vi "set units.vi"(8 "error in (no error)":errorcluster, 10 "Field Units (0: Gauss)":u16(ring) items=["Gauss", "Tesla", "Oersted", "Amp/meter"], 11 "VISA session":refnum<visa-resource-name>) -> (0 "error out":errorcluster, 3 "dup VISA session":refnum<visa-resource-name>)   [LabVIEW 2017]
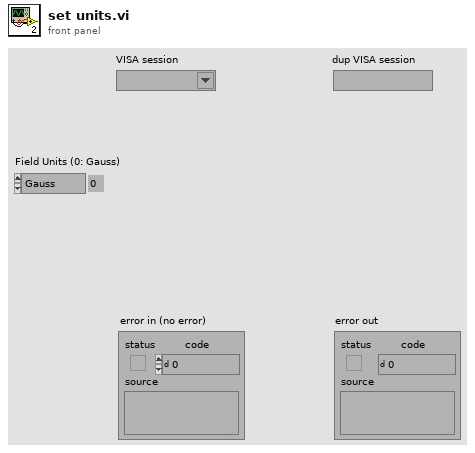
[diagram p1: front panel]
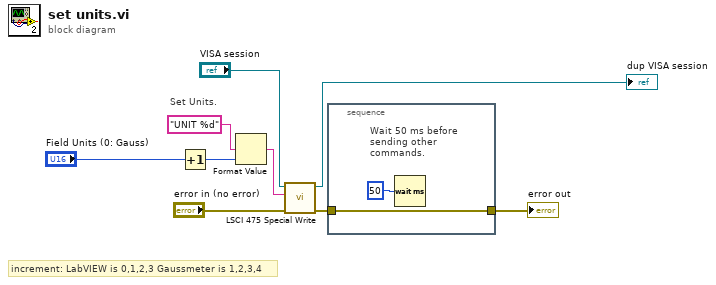
[diagram p0: block diagram]
diagram:
  # "increment: LabVIEW is 0,1,2,3 Gaussmeter is 1,2,3,4"
  # "Set Units."
  n1 = Increment(x="Field Units (0: Gauss)") -> (x+1=w3:u16)
  n2 = Format Value(format string="UNIT %d", value (0)=w3) -> (output string=w1:string)  [unwired: 1 in]
  n3 = call "LSCI 475 Special Write.vi"("error in (no error)"="error in (no error)", "Write Buffer (\"\")"=w1, "VISA session"="VISA session") -> ("error out"=w6:errorcluster, "dup VISA session"=→"dup VISA session":refnum<visa-resource-name>)  [unwired: 6 in, 1 out]
  n4 = stacked-sequence {
    tunnel: w6 -> [w10]
    tunnel: [w10] -> w7
    frame #0 {
      # "Wait 50 ms before\nsending other\ncommands."
      n5 = Wait (ms)(milliseconds to wait=u32 50) -> ()  [unwired: 1 out]
    }
  }
  "error out" <- w7
